vi "setup.vi"(8 "error in (no error)":errorcluster, 9 "Counter Refnums":T1, 10 "Counter Settings":T2 {"Array of Counter Settings"."Binwidth (ms)" format="%0.2f"}) -> (0 "error out":errorcluster, 3 "Counter out":refnum<class "Counter.lvclass">)   [LabVIEW 2013, in "Counter.lvclass"]
uses:
  Counter.lvclass
  Counter_Settings_Control.ctl
  counter_graph_refnums.ctl
  Counter.lvclass/Counter.ctl
  <vilib>/DAQmx/create/channels.llb/DAQmx Create Channel (CI-Count Edges).vi
  <vilib>/DAQmx/configure/timing.llb/DAQmx Timing (Sample Clock).vi
  <resource>/objmgr/daqmx.rc
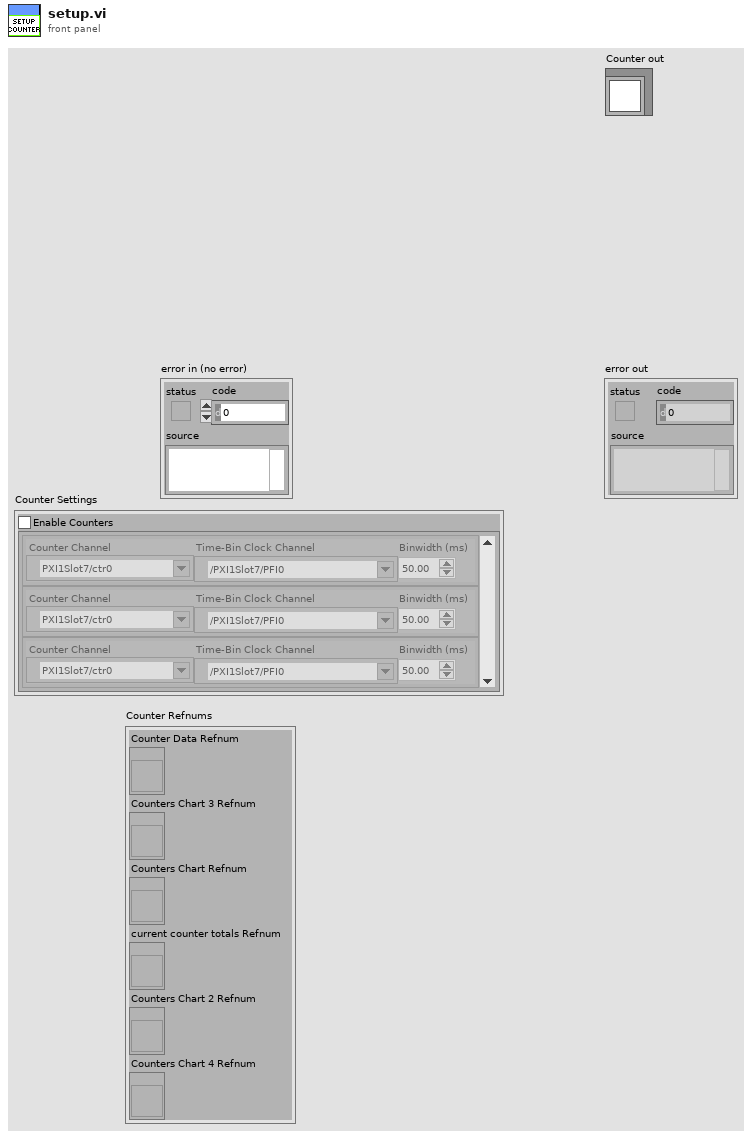
[diagram p1: front panel]
types:
  T1 = typedef "counter_graph_refnums.ctl" = cluster{"Counter Data Refnum":refnum<vi>, "Counters Chart 3 Refnum":refnum<vi>, "Counters Chart Refnum":refnum<vi>, "current counter totals Refnum":refnum<vi>, "Counters Chart 2 Refnum":refnum<vi>, "Counters Chart 4 Refnum":refnum<vi>}
  T2 = typedef "Counter.lvclass/Counter_Settings_Control.ctl" = cluster{"Enable Counters":bool, "Array of Counter Settings":cluster{"Counter Channel":tag, "Time-Bin Clock Channel":tag, "Binwidth (ms)":dbl}[]}
  T3 = cluster{"Counter Channel":tag, "Time-Bin Clock Channel":tag, "Binwidth (ms)":dbl}[]
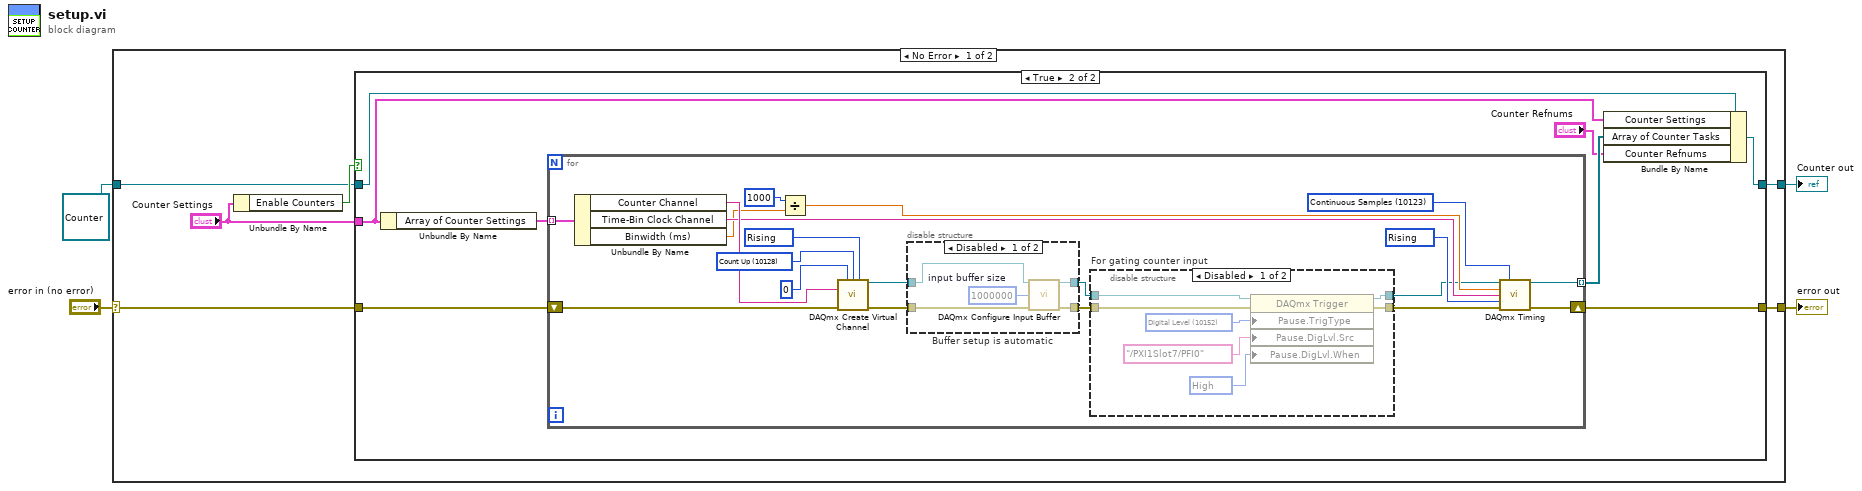
[diagram p0: block diagram]
diagram:
  n1 = case shown="No Error" "error in (no error)" {
    selector: "error in (no error)" -> [w8 w58]
    tunnel: [w9 w58] -> w3
    tunnel: [w6 w57] -> w1
    tunnel: refnum<class "Counter.lvclass"> refnum ("Counter in") -> [w7 w57]
    frame No Error {
      n2 = Unbundle By Name("Counter Settings") -> ("Enable Counters"=w10:bool)
      n3 = case shown="True" w10 {
        tunnel: w8 -> [w12 w20]
        tunnel: [w12 w19] -> w9
        tunnel: w7 -> [w11 w17]
        tunnel: [w11 w16] -> w6
        tunnel: "Counter Settings" -> [_ w14]
        frame False {
        }
        frame True {
          n4 = Unbundle By Name(w14) -> ("Array of Counter Settings"=w15:T3)
          n5 = for {
            tunnel: w15 -> [w40] mode=indexing
            shift-right: [w35] -> w19
            shift-left: w20 -> [w39]
            tunnel: [w34] -> w18 mode=indexing
            w29 = 10280 items=["Rising"=10280, "Falling"=10171] ("active edge")
            w30 = 10123 items=["Finite Samples"=10178, "Continuous Samples"=10123, "Hardware Timed Single Point"=12522] ("sample mode")
            w31 = 10280 items=["Rising"=10280, "Falling"=10171] ("edge")
            w32 = 10128 items=["Count Up"=10128, "Count Down"=10124, "Externally Controlled"=10326] ("count direction")
            n6 = Unbundle By Name(w40) -> ("Counter Channel"=w38:tag, "Time-Bin Clock Channel"=w37:tag, "Binwidth (ms)"=w36:dbl)
            n7 = Divide(x=1000, y=w36) -> (x/y=w26:dbl)
            n8 = call-poly <vilib>:"DAQmx Create Virtual Channel.vi"("initial count"=u32 0, "count direction"=w32, "edge"=w31, "counter"=w38, "error in"=w39) -> ("task out"=w28:refnum<k21>, "error out"=w27:errorcluster)  [unwired: 5 in, 4 out]
            n9 = disable-structure "Buffer setup is automatic" shown="Disabled" {
              disable-tunnel: w28 -> [w54 w55]
              disable-tunnel: w27 -> [w53 w56]
              disable-tunnel: [w52 w56] -> w23
              disable-tunnel: [w51 w55] -> w24
              frame Disabled {
                w50 = u32 1000000  # input buffer size
                n10 = call <vilib>:"DAQmx Configure Input Buffer.vi"("task/channels in"=w54, "buffer size (in samples per channel)"=w50, "error in"=w53) -> ("task out"=w51:refnum<k21>, "error out"=w52:errorcluster)  [unwired: 11 out]
              }
              frame Enabled {
              }
            }
            n11 = disable-structure "For gating counter input" shown="Disabled" {
              disable-tunnel: w24 -> [w47 w48]
              disable-tunnel: w23 -> [w46 w49]
              disable-tunnel: [w42 w48] -> w22
              disable-tunnel: [w41 w49] -> w21
              frame Disabled {
                w43 = 10152 items=["Analog Level"=10101, "Analog Window"=10103, "Digital Level"=10152, "Digital Pattern"=10398, "None"=10230] ("Pause.TrigType")
                w45 = 10192 items=["High"=10192, "Low"=10214] ("Pause.DigLvl.When")
                n12 = property class="DAQmx Trigger"(reference=w47, error in=w46, "Pause.TrigType"=w43, "Pause.DigLvl.Src"=tag "/PXI1Slot7/PFI0", "Pause.DigLvl.When"=w45) -> (reference out=w42:refnum<k21>, error out=w41:errorcluster)
              }
              frame Enabled {
              }
            }
            n13 = call-poly <vilib>:"DAQmx Timing.vi"("task/channels in"=w22, "sample mode"=w30, "rate"=w26, "source"=w37, "active edge"=w29, "error in"=w21) -> ("task out"=w34:refnum<k21>, "error out"=w35:errorcluster)  [unwired: 1 in, 7 out]
          }
          n14 = Bundle By Name(cluster=w17, "Counter Settings"=w14, "Array of Counter Tasks"=w18, "Counter Refnums"="Counter Refnums") -> (w16:refnum<class "Counter.lvclass">)
        }
      }
    }
    frame Error {
    }
  }
  "error out" <- w3
  "Counter out" <- w1
